vi "Test_Benchmarking_ManyLocalLogEventCall_AvgCallTimeSub10uS.vi"(8 "error in (no error)":errorcluster, 11 "Benchmarking in":refnum<class "Benchmarking.lvclass">) -> (0 "error out":errorcluster, 3 "Benchmarking out":refnum<class "Benchmarking.lvclass">)   [LabVIEW 2017, in "Benchmarking.lvclass"]
uses:
  Benchmarking.lvclass
  Source/LVQueue Sink/LVQueue Sink.lvclass/LVQueue Sink.ctl
  Source/Composed Log/LoggerReference/LoggerReference.lvclass/LoggerReference.ctl
  0fe8a2ce-6c26-4d19-a6a0-eb7461585297.vi
  <vilib>/Analysis/baseanly.llb/Mean (DBL).vi
  Source/Composed Log/LoggerReference/Return Aggregate Queues.vi
  Source/Composed Log/LoggerReference/Add Aggregate Log.vi
  0fe8a2ce-6c26-4d19-a6a0-eb7461585297.vi/f88a3b2e-b24f-4764-a520-80cd8d0ee0ad.vi
  Source/Composed Log/LoggerReference/Send Add Sink.vi
  Source/LVQueue Sink/LVQueue Sink.lvclass
  C:/CS/Internal/LabVIEW/Logger/Source/Composed Log/Log Sink/Log Sink.lvclass
  Source/Composed Log/Application Logger/Launch Worker Loop.vi
  Source/Composed Log/LoggerReference/Initialize Logger Instance.vi
  Source/Composed Log/LoggerReference/LoggerReference.lvclass
  Source/Composed Log/IErrorFormat/IErrorFormat.lvclass
  Source/Composed Log/Log Sink/Log Sink.lvclass
  <vilib>/Analysis/NI_AALBase.lvlib
  <vilib>/addons/_JKI Toolkits/VI Tester/TestCase.llb/TestCase.lvclass
  C:/Program Files (x86)/National Instruments/LabVIEW 2017/vi.lib/addons/_JKI Toolkits/VI Tester/TestCase.llb/TestCase.lvclass
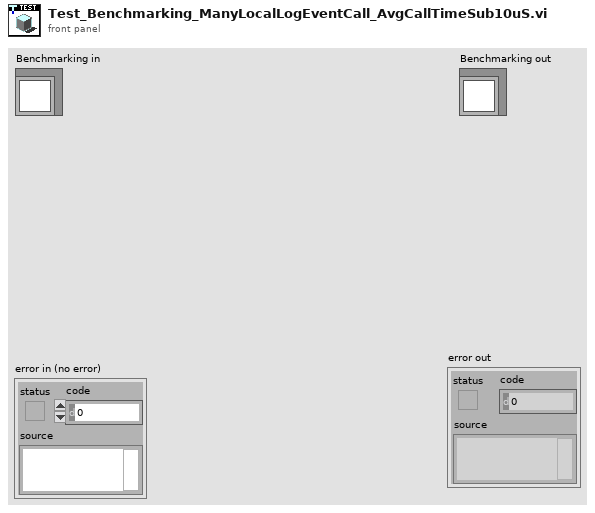
[diagram p1: front panel]
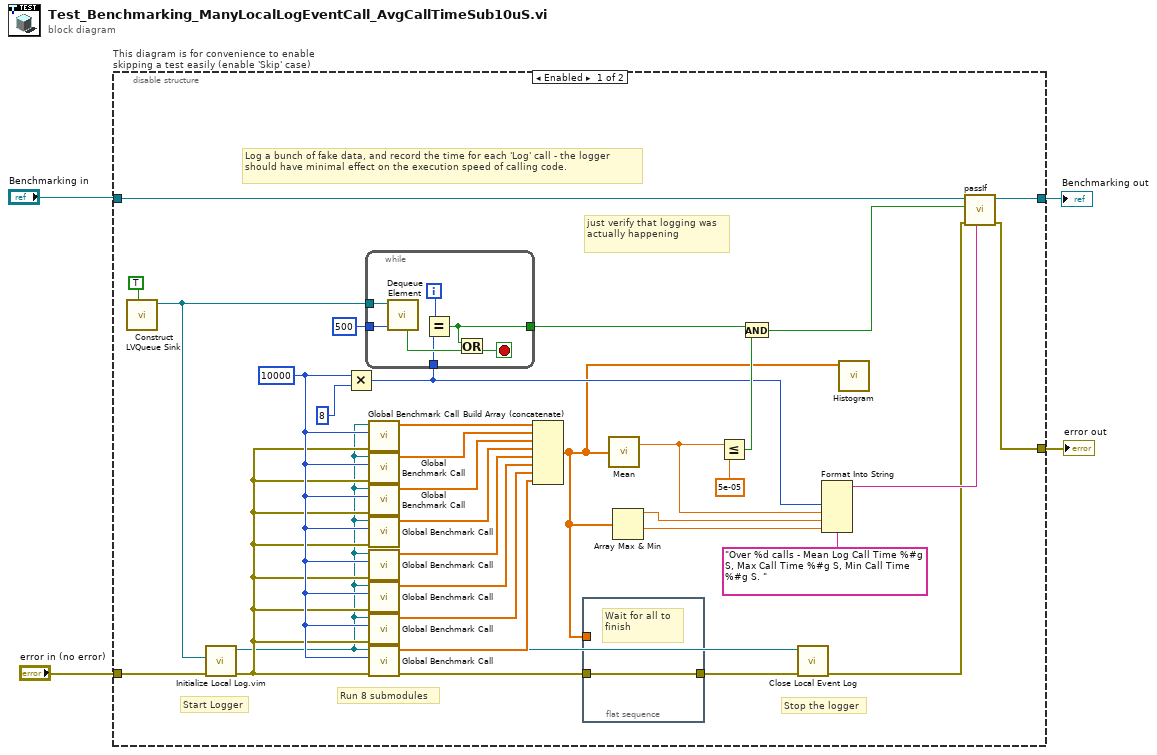
[diagram p0: block diagram]
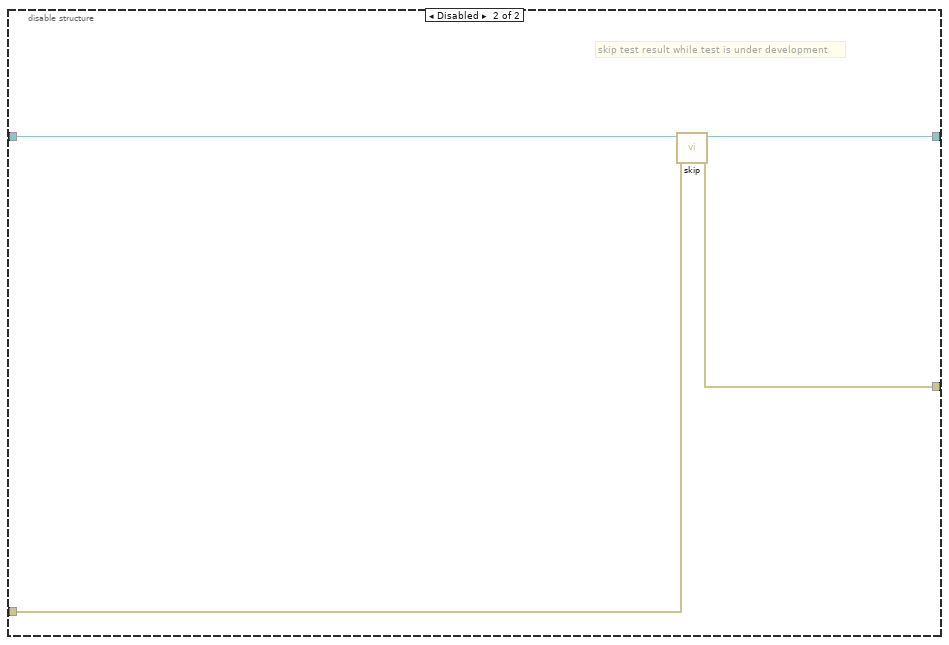
[diagram p2: hidden frame]
diagram:
  n1 = disable-structure "This diagram is for convenience to enable skipping a test easily (enable 'Skip' case)" shown="Enabled" {
    disable-tunnel: "Benchmarking in" -> [w36 w49]
    disable-tunnel: [w35 w47] -> w4
    disable-tunnel: [w37 w48] -> w3
    disable-tunnel: "error in (no error)" -> [w11 w46]
    frame Enabled {
      w19 = 10000 ("Count")
      # "just verify that logging was actually happening"
      # "Run 8 submodules"
      # "Stop the logger"
      # "Start Logger"
      # "Log a bunch of fake data, and record the time for each 'Log' call - the logger should have minimal effect on the execution speed of calling code."
      n2 = call "Construct LVQueue Sink.vi"("User Shutdown? (F)"=TRUE) -> ("LVQueue Sink out"=w10:refnum<class "LVQueue Sink.lvclass">)  [unwired: 9 in, 1 out]
      n3 = call "Initialize Local Log.vim"("error in (no error)"=w11, "Startup Sink(s)"=w10) -> ("error out"=w9:errorcluster, "Log Instance Reference"=w8:refnum<class "LoggerReference.lvclass">)  [unwired: 7 in, 1 out]
      n4 = Multiply(x=w19, y=8 ("x")) -> (x*y=w6:i32)
      n5 = while {
        tunnel: w10 -> [w45]
        tunnel: w6 -> [w43]
        tunnel: [w39] -> w16
        tunnel: 500 ("timeout in ms (-1)") -> [w40]
        i -> [w42]
        stop <- w41 stop-if-true
        n6 = call "Dequeue Element.vi"("timeout in ms (-1)"=w40, "LVQueue Sink in"=w45) -> ("Timed Out?"=w44:bool)  [unwired: 6 in, 3 out]
        n7 = Equal?(x=w42, y=w43) -> (x = y?=w39:bool)
        n8 = Or(x=w39, y=w44) -> (x .or. y?=w41:bool)
      }
      n9 = call "Global Benchmark Call.vi"("error in"=w9, "Count"=w19, "Log Instance"=w8) -> ("Call Times"=w28:dbl[])  [unwired: 7 in, 1 out]
      n10 = call "Global Benchmark Call.vi"("error in"=w9, "Count"=w19, "Log Instance"=w8) -> ("Call Times"=w27:dbl[])  [unwired: 7 in, 1 out]
      n11 = call "Global Benchmark Call.vi"("error in"=w9, "Count"=w19, "Log Instance"=w8) -> ("Call Times"=w26:dbl[])  [unwired: 7 in, 1 out]
      n12 = call "Global Benchmark Call.vi"("error in"=w9, "Count"=w19, "Log Instance"=w8) -> ("Call Times"=w25:dbl[])  [unwired: 7 in, 1 out]
      n13 = call "Global Benchmark Call.vi"("error in"=w9, "Count"=w19, "Log Instance"=w8) -> ("Call Times"=w24:dbl[])  [unwired: 7 in, 1 out]
      n14 = call "Global Benchmark Call.vi"("error in"=w9, "Count"=w19, "Log Instance"=w8) -> ("Call Times"=w23:dbl[])  [unwired: 7 in, 1 out]
      n15 = call "Global Benchmark Call.vi"("error in"=w9, "Count"=w19, "Log Instance"=w8) -> ("Call Times"=w22:dbl[])  [unwired: 7 in, 1 out]
      n16 = call "Global Benchmark Call.vi"("error in"=w9, "Count"=w19, "Log Instance"=w8) -> ("error out"=w14:errorcluster, "Call Times"=w21:dbl[])  [unwired: 7 in]
      n17 = Build Array (concatenate)(w28, w27, w26, w25, w24, w23, w22, w21) -> (w5:dbl[])
      n18 = flat-sequence {
        tunnel: w5 -> [_]
        tunnel: w14 -> [w38]
        tunnel: [w38] -> w13
        frame #0 {
          # "Wait for all to finish"
        }
      }
      n19 = call-poly <vilib>:"Mean.vi"("X"=w5) -> ("mean"=w7:dbl)  [unwired: 1 out]
      n20 = Array Max & Min(array=w5) -> (max value=w31:dbl, min value=w30:dbl)  [unwired: 2 out]
      n21 = Less Or Equal?(x=w7, y=5e-05) -> (x <= y?=w33:bool)
      n22 = And(x=w16, y=w33) -> (x .and. y?=w17:bool)
      n23 = call "Close Local Event Log.vi"("error in (no error)"=w13, "Log Instance"=w8) -> ("error out"=w12:errorcluster)  [unwired: 9 in]
      n24 = Format Into String(format string="Over %d calls - Mean Log Call Time %#g S, Max Call Time %#g S, Min Call Time %#g S. ", w6, w7, w31, w30) -> (resulting string=w29:string)  [unwired: 2 in, 1 out]
      n25 = call <vilib>:"Histogram.vi"("X"=w5) -> ()  [unwired: 7 in, 4 out]
      n26 = call-dynamic "passIf.vi"("custom report message (\"\")"=w29, "error in (no error)"=w12, "pass"=w17, "TestCase in"=w36) -> ("error out"=w37:errorcluster, "TestCase out"=w35:refnum<class "Benchmarking.lvclass">)  [unwired: 6 in]
    }
    frame Disabled {
      # "skip test result while test is under development"
      n27 = call <vilib>:"skip.vi"("error in (no error)"=w46, "TestCase in"=w49) -> ("error out"=w48:errorcluster, "TestCase out"=w47:refnum<class "Benchmarking.lvclass">)  [unwired: 8 in]
    }
  }
  "error out" <- w3
  "Benchmarking out" <- w4
